vi "Post VI Refnum.vi"(8 "error in (no error)":errorcluster, 11 "Controller Template in":refnum<class "DataLoggerUI.lvclass">) -> (0 "error out":errorcluster, 3 "Controller Template out":refnum<class "DataLoggerUI.lvclass">)   [LabVIEW 2020, in "DataLogger.lvlib" / "DataLoggerUI.lvlib" / "DataLoggerUI.lvclass"]
uses:
  DataLoggerUI.lvclass
  C:/Program Files/National Instruments/LabVIEW 2020/vi.lib/ActorFramework/Actor/Actor.lvclass
  <vilib>/ActorFramework/Actor/Actor.lvclass/Actor.ctl
  DataLoggerUI.lvclass/DataLoggerUI.ctl
  Interface/DockingDevice Messages/PostUserInterfaceRefnum Msg/PostUserInterfaceRefnum Msg.lvclass/PostUserInterfaceRefnum Msg.ctl
  <vilib>/ActorFramework/Message Enqueuer/Message Enqueuer.lvclass/Message Enqueuer.ctl
  <vilib>/ActorFramework/Message Enqueuer/Enqueue.vi
  Interface/DockingDevice Messages/PostUserInterfaceRefnum Msg/PostUserInterfaceRefnum Msg.lvclass
  C:/Program Files/National Instruments/LabVIEW 2020/vi.lib/ActorFramework/Message/Message.lvclass
  <vilib>/ActorFramework/Message Priority Queue/Priority Enqueue.vi
  <vilib>/ActorFramework/Actor/Actor.lvclass
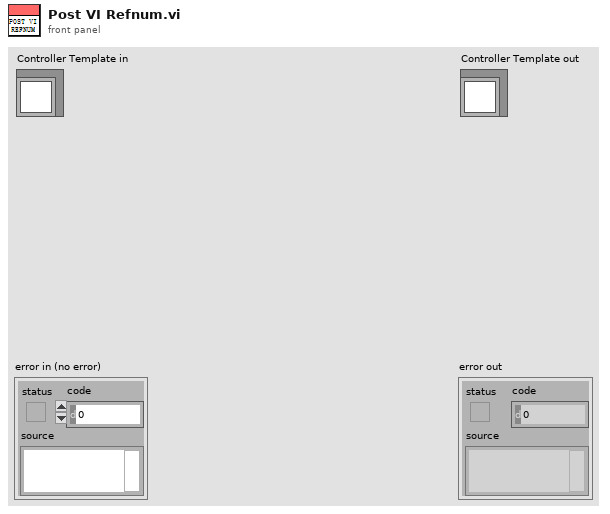
[diagram p1: front panel]
types:
  T1 = enum32{"Invalid", "Standard", "Closed", "Hidden", "Minimized", "Maximized"}
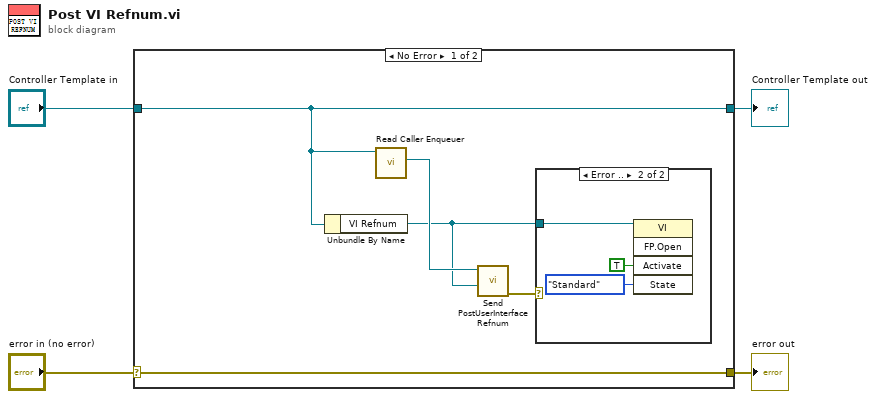
[diagram p0: block diagram]
diagram:
  n1 = case shown="No Error" "error in (no error)" {
    selector: "error in (no error)" -> [w9 w14]
    tunnel: [w9 w14] -> w3
    tunnel: [w7 w13] -> w1
    tunnel: "Controller Template in" -> [w7 w13]
    frame No Error {
      n2 = Unbundle By Name(w7) -> ("VI Refnum"=w5:refnum<vi>)
      n3 = call <vilib>:"Read Caller Enqueuer.vi"("Actor"=w7) -> ("Caller Enqueuer"=w8:refnum<class "Message Enqueuer.lvclass">)  [unwired: 10 in]
      n4 = call "Send PostUserInterfaceRefnum.vi"("VI Refnum"=w5, "Message Enqueuer"=w8) -> ("error out"=w6:errorcluster)  [unwired: 8 in, 1 out]
      n5 = case shown="Error .." w6 {
        tunnel: w5 -> [_ w12]
        frame No Error {
        }
        frame Error {
          n6 = invoke class="VI" method="FP.Open"(reference=w12, "Activate"=TRUE ("Activate?"), "State"=T1."Standard") -> ()  [unwired: 2 in, 5 out]
        }
      }
    }
    frame Error {
    }
  }
  "error out" <- w3
  "Controller Template out" <- w1
